vi "Create JSON Lexer.vi"(8 "error in (no error)":errorcluster) -> (0 "error out":errorcluster, 3 "JSON Lexer":refnum<class "JSON Lexer.lvclass">)   [LabVIEW 2019, in "JKI JSON Serialization.lvlib" / "JSON Lexer.lvclass"]
doc: "JKI JSON 1.1.10.37\nTomi Maila - JKI\nCopyright (c) 2017, JKI"
uses:
  JSON Lexer.lvclass
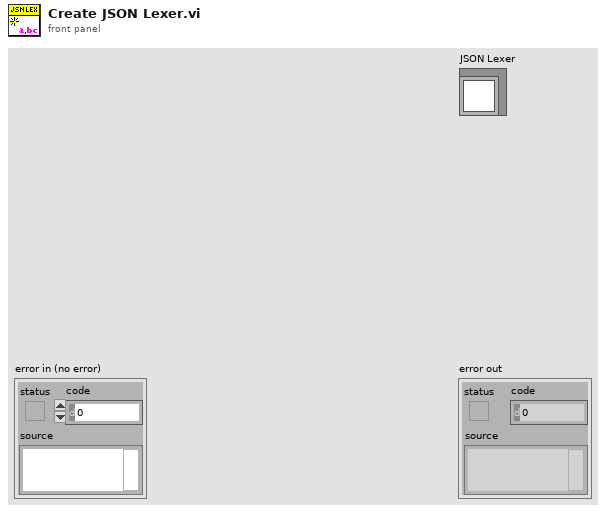
[diagram p1: front panel]
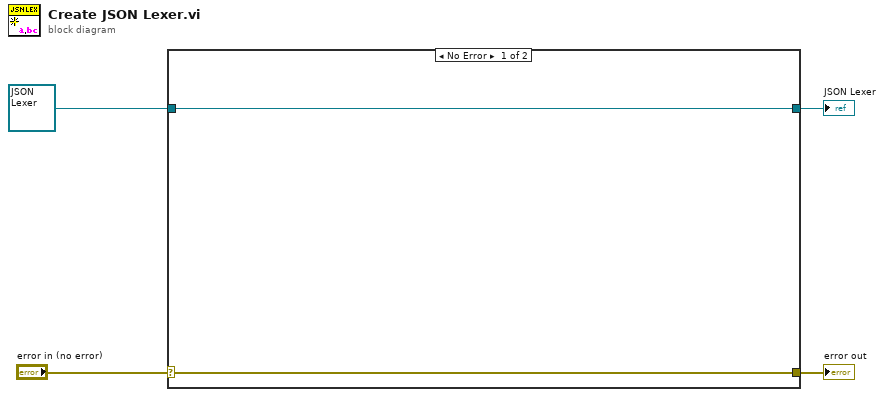
[diagram p0: block diagram]
diagram:
  n1 = case shown="No Error" "error in (no error)" {
    selector: "error in (no error)" -> [w5 w8]
    tunnel: [w5 w8] -> w3
    tunnel: [w6 w7] -> w1
    tunnel: refnum<class "JSON Lexer.lvclass"> refnum ("JSON Lexer in") -> [w6 w7]
    frame No Error {
    }
    frame Error {
    }
  }
  "error out" <- w3
  "JSON Lexer" <- w1
